vi "AlliGator Save FLI Dataset Gates to HDF5 (VDM).vi"(4 "Channel 2 Gate Image Array":T2[](array[typedef]), 6 "Channel 1 Gate Image Array":T2[](array[typedef]), 7 "replace?":bool, 8 "error in (no error)":errorcluster, 10 "Gate Names":string[](array[string]), 11 "HDF5 File ref in":T1 format="%.0x") -> (0 "error out":errorcluster, 3 "HDF5 File ref out":T1 format="%.0x")   [LabVIEW 2021, in "AlliGator Files.lvlib"]
doc: "Saves gate images (single- or dual-channel) to HDF5 file."
uses:
  AlliGator Files.lvlib
  <vilib>/addons/h5labview2/base/hid_t.ctl
  <vilib>/vision/Image Controls.llb/IMAQ Image.ctl
  AlliGator Abort.vi
  <vilib>/Utility/error.llb/Error Cluster From Error Code.vi
  <vilib>/ErrorRing/Error Ring.xnode
  <vilib>/addons/h5labview2/group/H5G.lvlib
  GUI/GUI.lvlib
  AlliGator Globals, Variables & Constants.lvlib
panel:
  # "see the AlliGator License on the block diagram (Ctrl+E or Window:Show Block Diagram)"
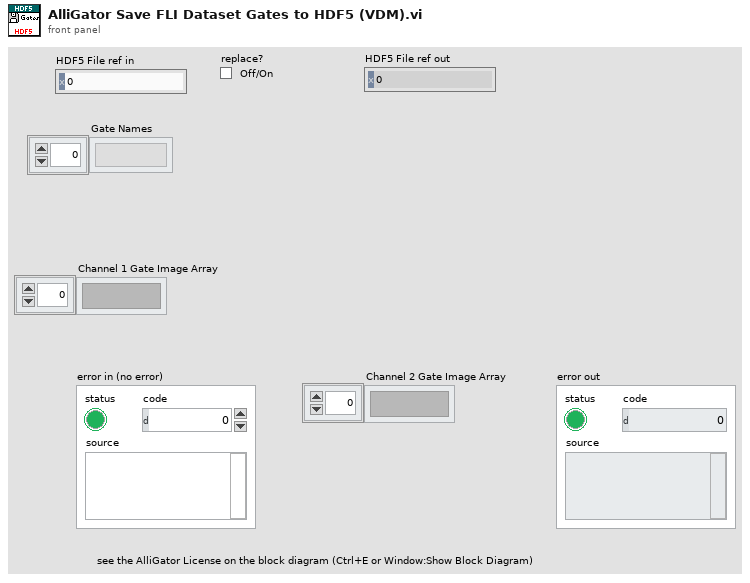
[diagram p1: front panel]
types:
  T1 = typedef "hid_t.ctl" = i64
  T2 = typedef "IMAQ Image.ctl" = refnum<image>
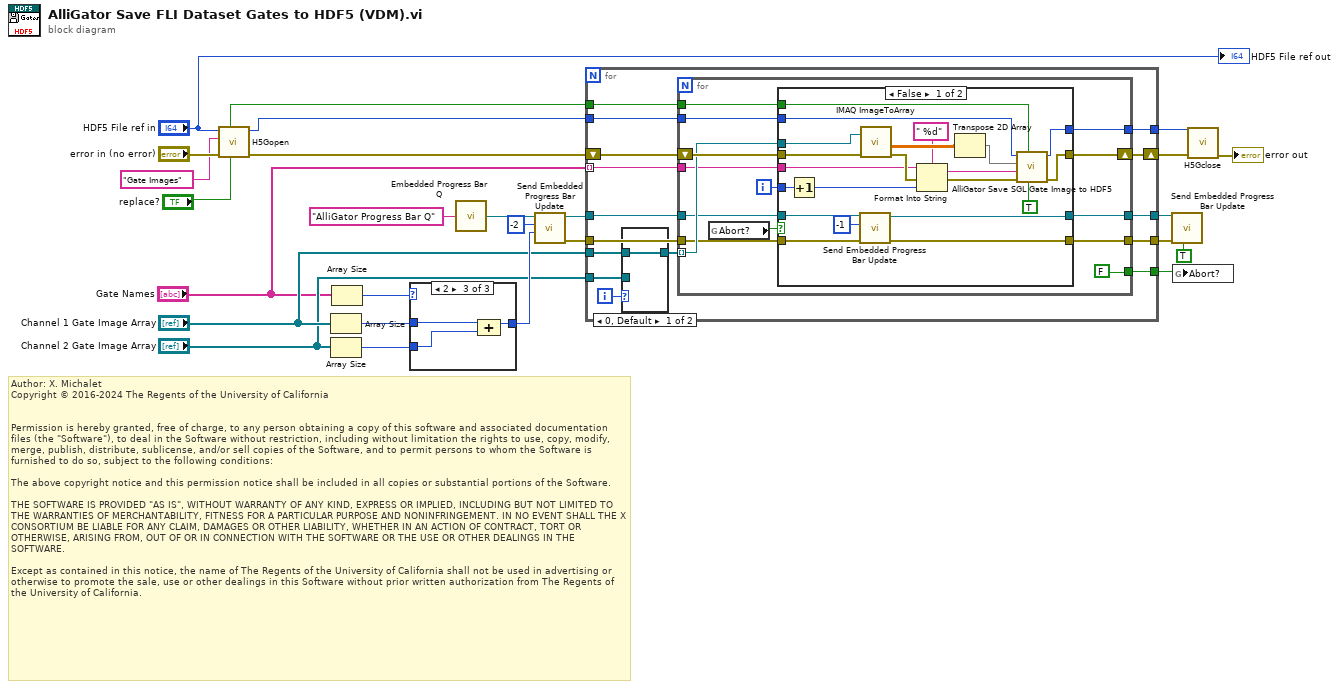
[diagram p0: block diagram]
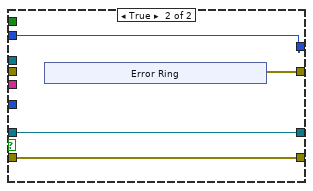
[diagram p3: hidden frame]
diagram:
  # "Author: X. Michalet\nCopyright © 2016-2024 The Regents of the University of California\n \n\nPermission is hereby granted, free of charge, to any person obtaining a copy of this software and associated documentation files (the \"Software\"), to deal in the Software without restriction, including without limitation the rights to use, copy, modify, merge, publish, distribute, sublicense, and/or sell copies of the Software, and to permit persons to whom the Software is furnished to do so, subject to the following conditions:\n\nThe above copyright notice and this permission notice shall be included in all copies or substantial portions of the Software.\n\nTHE SOFTWARE IS PROVIDED \"AS IS\", WITHOUT WARRANTY OF ANY KIND, EXPRESS OR IMPLIED, INCLUDING BUT NOT LIMITED TO THE WARRANTIES OF MERCHANTABILITY, FITNESS FOR A PARTICULAR PURPOSE AND NONINFRINGEMENT. IN NO EVENT SHALL THE X CONSORTIUM BE LIABLE FOR ANY CLAIM, DAMAGES OR OTHER LIABILITY, WHETHER IN AN ACTION OF CONTRACT, TORT OR OTHERWISE, ARISING FROM, OUT OF OR IN CONNECTION WITH THE SOFTWARE OR THE USE OR OTHER DEALINGS IN THE SOFTWARE.\n\nExcept as contained in this notice, the name of The Regents of the University of California shall not be used in advertising or otherwise to promote the sale, use or other dealings in this Software without prior written authorization from The Regents of the University of California."
  n1 = call <vilib>:"H5Gopen.vi"("create? (F)"="replace?", "error in (no error)"="error in (no error)", "name"="Gate Images", "ref in"="HDF5 File ref in") -> ("error out"=w1:errorcluster, "group out"=w8:T1)  [unwired: 6 in]
  n2 = Array Size(array="Channel 1 Gate Image Array") -> (size(s)=w4:i32)
  n3 = Array Size(array="Channel 2 Gate Image Array") -> (size(s)=w3:i32)
  n4 = Array Size(array="Gate Names") -> (size(s)=w23:i32)
  n5 = case shown="2" w23 {
    tunnel: [w26 w27 w30] -> w22
    tunnel: w4 -> [w26 w27 w29]
    tunnel: w3 -> [_ _ w28]
    frame 0, Default {
    }
    frame 1 {
    }
    frame 2 {
      n6 = Compound Arithmetic op=ADD(w29, w28) -> (w30:i32)
    }
  }
  n7 = call "Embedded Progress Bar Q.vi"("Progress Bar Queue Name"="AlliGator Progress Bar Q") -> ("Progress Bar Queue"=w19:refnum<queue>)  [unwired: 6 in]
  n8 = call "Send Embedded Progress Bar Update.vi"("Max Iterations N"=w22, "Current Iteration i (i or -1: standard or || iteration; 0 or -2: first standard or || iteration)"=-2 ("Current Iteration i (-1: || iteration, -2: first || iteration)"), "Progress Bar Queue in"=w19) -> ("Error Out"=w21:errorcluster, "Progress Bar Queue out"=w20:refnum<queue>)  [unwired: 7 in]
  n9 = for {
    tunnel: "Channel 1 Gate Image Array" -> [w33]
    tunnel: "Gate Names" -> [w35] mode=indexing
    shift-right: [w43] -> w10
    shift-left: w1 -> [w44]
    tunnel: w20 -> [w37]
    tunnel: [w40] -> w14
    tunnel: w21 -> [w36]
    tunnel: [w38] -> w17
    tunnel: "replace?" -> [w41]
    tunnel: [w39] -> w16
    tunnel: w8 -> [w45]
    tunnel: [w42] -> w11
    tunnel: "Channel 2 Gate Image Array" -> [w31]
    i -> [w34]
    n10 = case shown="0, Default" w34 {
      tunnel: w33 -> [w46 _]
      tunnel: [w46 w47] -> w32
      tunnel: w31 -> [_ w47]
      frame 0, Default {
      }
      frame 1 {
      }
    }
    n11 = for {
      tunnel: w32 -> [w60] mode=indexing
      shift-right: [w58] -> w43
      shift-left: w44 -> [w61]
      tunnel: w41 -> [w55]
      tunnel: w45 -> [w57]
      tunnel: [w56] -> w42
      tunnel: w37 -> [w53]
      tunnel: [w52] -> w40
      tunnel: [FALSE ("Abort?")] -> w39
      tunnel: [w50] -> w38
      tunnel: w36 -> [w49]
      tunnel: w35 -> [w48]
      i -> [w59]
      n12 = global read "AlliGator Abort.vi" "Abort?"() -> (w54:bool)
      n13 = case shown="False" w54 {
        tunnel: w61 -> [w82 _]
        tunnel: w60 -> [w81 _]
        tunnel: w59 -> [w67 _]
        tunnel: [w74 w85] -> w58
        tunnel: w57 -> [w73 w86]
        tunnel: [w72 w86] -> w56
        tunnel: w55 -> [w71 _]
        tunnel: w53 -> [w69 w84]
        tunnel: [w68 w84] -> w52
        tunnel: [w66 w83] -> w50
        tunnel: w49 -> [w64 w83]
        tunnel: w48 -> [w63 _]
        frame False {
          n14 = Increment(x=w67) -> (x+1=w80:i32)
          n15 = call "Send Embedded Progress Bar Update.vi"("Error In"=w64, "Current Iteration i (i or -1: standard or || iteration; 0 or -2: first standard or || iteration)"=-1 ("Current Iteration i (i or -1: standard or || iteration; 0 or -2: first standard or || iteration)"), "Progress Bar Queue in"=w69) -> ("Error Out"=w66:errorcluster, "Progress Bar Queue out"=w68:refnum<queue>)  [unwired: 7 in]
          n16 = call "IMAQ ImageToArray"("error in (no error)"=w82, "Image"=w81) -> ("Image Pixels (Float)"=w77:sgl[][], "error out"=w75:errorcluster)  [unwired: 2 in, 3 out]
          n17 = Format Into String(format string=" %d", initial string=w63, error in=w75, w80) -> (resulting string=w79:string, error out=w78:errorcluster)
          n18 = Transpose 2D Array(2D array=w77) -> (transposed array=w70:sgl[][])
          n19 = call "AlliGator Save SGL Gate Image to HDF5.vi"("Compression"=TRUE, "Replace?"=w71, "error in (no error)"=w78, "Image Name"=w79, "Data"=w70, "ref in"=w73) -> ("error out"=w74:errorcluster, "ref out"=w72:T1)  [unwired: 4 in]
        }
        frame True {
          n20 = xnode "Error Ring"() -> ("error out"=w85:errorcluster)
        }
      }
    }
  }
  n21 = call "Send Embedded Progress Bar Update.vi"("Stop Progress Bar (F)"=TRUE, "Error In"=w17, "Progress Bar Queue in"=w14) -> ()  [unwired: 7 in, 2 out]
  n22 = global write "AlliGator Abort.vi" "Abort?"(w16) -> ()
  n23 = call <vilib>:"H5Gclose.vi"("error in (no error)"=w10, "group in"=w11) -> ("error out"=→"error out":errorcluster)  [unwired: 9 in]
  "HDF5 File ref out" <- "HDF5 File ref in"
